vi "GetFovRayData.vi"(6 "Sensor position":cluster{"X":sgl, "Y":sgl, "Z":sgl}={"X"=0.0, "Y"=0.0, "Z"=70.75}, 8 "Max distance":dbl, 9 "Kinect FOV (deg)":cluster{"Height":i32, "Width":i32}, 10 "Sensor Yaw angle (deg)":dbl, 11 "Elevation Angle":i32) -> (3 "Planes":T1)   [LabVIEW 2014]
uses:
  <vilib>/Math Plots/3D Math Plots/3D Scatter/3D Scatter XCtrl/3D Scatter.xctl
  <vilib>/Math Plots/3D Math Plots/3D Plot/3D Plot Datatype/3D Plot Datatype.lvclass
  <vilib>/Math Plots/3D Math Plots/3D Scatter/3D Scatter Datatype/Public/Plot Helper (Vector).vi
  <vilib>/Analysis/coordinate.llb/3D Coordinate Conversion (Array).vi
  <vilib>/Analysis/NI_AALPro.lvlib
  <vilib>/Math Plots/3D Math Plots/3D Scatter/3D Scatter Datatype/3D Scatter Datatype.lvclass
panel:
  out "3D Scatter":refnum<class "3D Plot Datatype.lvclass">[](xcontrol)
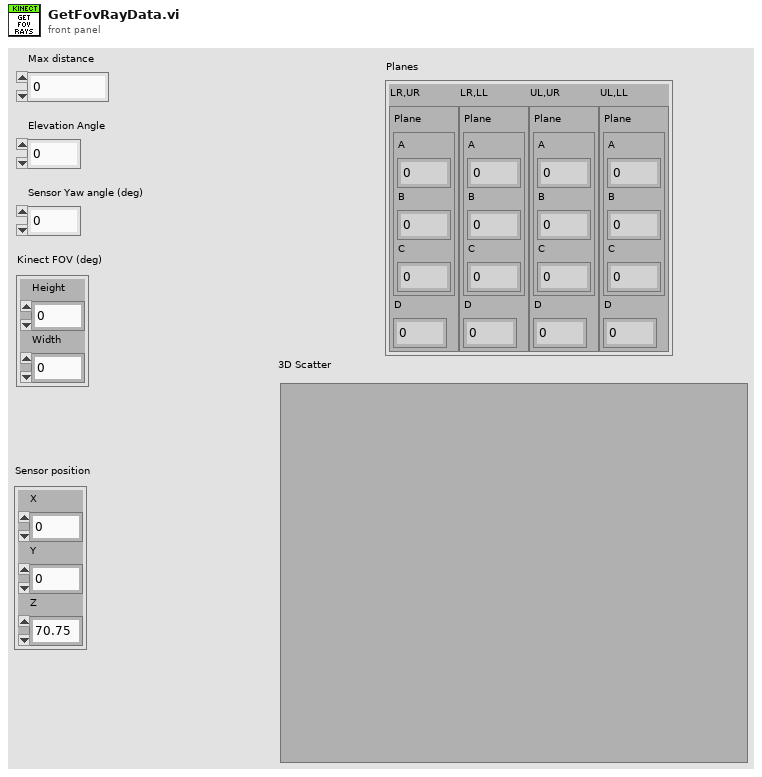
[diagram p1: front panel]
types:
  T1 = cluster{"LR,UR":cluster{"Plane":cluster{"A":dbl, "B":dbl, "C":dbl}, "D":dbl}, "LR,LL":cluster{"Plane":cluster{"A":dbl, "B":dbl, "C":dbl}, "D":dbl}, "UL,UR":cluster{"Plane":cluster{"A":dbl, "B":dbl, "C":dbl}, "D":dbl}, "UL,LL":cluster{"Plane":cluster{"A":dbl, "B":dbl, "C":dbl}, "D":dbl}}
  T2 = cluster{"Numeric":dbl, "Numeric":dbl, "Numeric":dbl}[]
  T3 = cluster{"Numeric":dbl, "Numeric":dbl, "Numeric":dbl}
  T4 = cluster{"Sensor position":cluster{"X":sgl, "Y":sgl, "Z":sgl}, cluster{"Numeric":dbl, "Numeric":dbl, "Numeric":dbl}, cluster{"Numeric":dbl, "Numeric":dbl, "Numeric":dbl}}
  T5 = cluster{"Plane":cluster{"A":dbl, "B":dbl, "C":dbl}, "D":dbl}
  T6 = cluster{"[0]":cluster{"Plane":cluster{"A":dbl, "B":dbl, "C":dbl}, "D":dbl}, "[1]":cluster{"Plane":cluster{"A":dbl, "B":dbl, "C":dbl}, "D":dbl}, "[2]":cluster{"Plane":cluster{"A":dbl, "B":dbl, "C":dbl}, "D":dbl}, "[3]":cluster{"Plane":cluster{"A":dbl, "B":dbl, "C":dbl}, "D":dbl}}
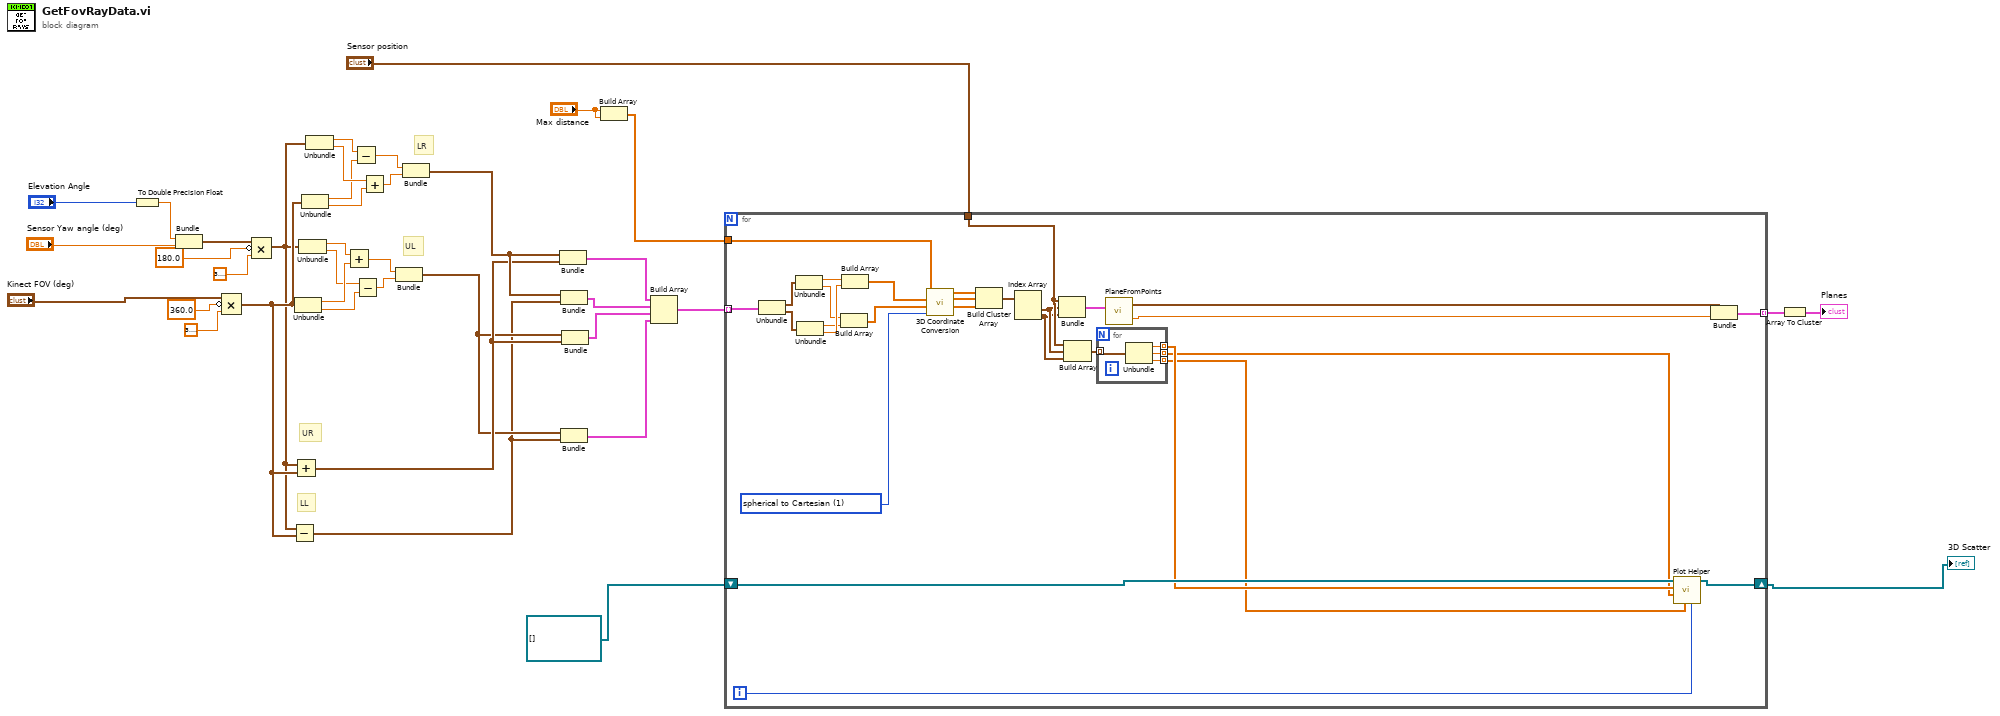
[diagram p0: block diagram]
diagram:
  # "LL"
  # "UR"
  # "UL"
  # "LR"
  n1 = To Double Precision Float(number="Elevation Angle") -> (double precision float=w37:dbl)
  n2 = Bundle(w37, "Sensor Yaw angle (deg)"="Sensor Yaw angle (deg)") -> (w36:cluster{dbl, "Sensor Yaw angle (deg)":dbl})  [unwired: 1 in]
  n3 = Compound Arithmetic op=MULTIPLY("Kinect FOV (deg)", invert 360.0 ("value"), 3.141592653589793) -> (w18:cluster{"Height":dbl, "Width":dbl})
  n4 = Compound Arithmetic op=MULTIPLY(w36, invert 180.0 ("value"), 3.141592653589793) -> (w17:cluster{dbl, "Sensor Yaw angle (deg)":dbl})
  n5 = Subtract(x=w17, y=w18) -> (x-y=w13:cluster{dbl, dbl})
  n6 = Add(x=w17, y=w18) -> (x+y=w15:cluster{dbl, dbl})
  n7 = Unbundle(w18) -> ("Height"=w29:dbl, "Width"=w27:dbl)
  n8 = Unbundle(w17) -> (w30:dbl, "Sensor Yaw angle (deg)"=w28:dbl)
  n9 = Unbundle(w18) -> ("Height"=w20:dbl, "Width"=w22:dbl)
  n10 = Unbundle(w17) -> (w19:dbl, "Sensor Yaw angle (deg)"=w21:dbl)
  n11 = Add(x=w30, y=w29) -> (x+y=w25:dbl)
  n12 = Subtract(x=w19, y=w20) -> (x-y=w24:dbl)
  n13 = Subtract(x=w28, y=w27) -> (x-y=w26:dbl)
  n14 = Add(x=w21, y=w22) -> (x+y=w23:dbl)
  n15 = Bundle(w25, w26) -> (w14:cluster{dbl, dbl})  [unwired: 1 in]
  n16 = Bundle(w24, w23) -> (w16:cluster{dbl, dbl})  [unwired: 1 in]
  n17 = Bundle(w16, w15) -> (w12:cluster{cluster{dbl, dbl}, cluster{dbl, dbl}})  [unwired: 1 in]
  n18 = Bundle(w16, w13) -> (w11:cluster{cluster{dbl, dbl}, cluster{dbl, dbl}})  [unwired: 1 in]
  n19 = Bundle(w14, w13) -> (w10:cluster{cluster{dbl, dbl}, cluster{dbl, dbl}})  [unwired: 1 in]
  n20 = Bundle(w14, w15) -> (w9:cluster{cluster{dbl, dbl}, cluster{dbl, dbl}})  [unwired: 1 in]
  n21 = Build Array("Max distance", "Max distance") -> (w6:dbl[])
  n22 = Build Array(w12, w11, w9, w10) -> (w8:cluster{cluster{dbl, dbl}, cluster{dbl, dbl}}[])
  n23 = for {
    tunnel: w8 -> [w67] mode=indexing
    tunnel: w6 -> [w60]
    tunnel: "Sensor position" -> [w53]
    tunnel: [w57] -> w4 mode=indexing
    shift-right: [w46] -> w1
    shift-left: refnum<class "3D Plot Datatype.lvclass">[] [] ("3D Plot lvclass Array out") -> [w47]
    i -> [w42]
    w68 = u16 1 items=["Cartesian to spherical", "spherical to Cartesian", "Cartesian to cylindrical", "cylindrical to Cartesian", "spherical to cylindrical", "cylindrical to spherical"] ("conversion type")
    n24 = Unbundle(w67) -> (w66:cluster{dbl, dbl}, w65:cluster{dbl, dbl})
    n25 = Unbundle(w66) -> (w64:dbl, w61:dbl)
    n26 = Unbundle(w65) -> (w62:dbl, w63:dbl)
    n27 = Build Array(w61, w62) -> (w40:dbl[])
    n28 = Build Array(w64, w63) -> (w41:dbl[])
    n29 = call-poly <vilib>:"3D Coordinate Conversion.vi"("conversion type"=w68, "Axis 3"=w40, "Axis 2"=w41, "Axis 1"=w60) -> ("Axis 3 Out"=w54:dbl[], "Axis 2 Out"=w56:dbl[], "Axis 1 Out"=w55:dbl[])  [unwired: 4 in, 1 out]
    n30 = Build Cluster Array(w55, w56, w54) -> (w59:T2)
    n31 = Index Array(array=w59) -> (element #1=w52:T3, element #2=w51:T3)  [unwired: 2 in]
    n32 = Bundle("Sensor position"=w53, w52, w51) -> (w58:T4)  [unwired: 1 in]
    n33 = Build Array(w53, w52, w51) -> (w50:T2)
    n34 = for {
      tunnel: w50 -> [w72] mode=indexing
      tunnel: [w71] -> w45 mode=indexing
      tunnel: [w70] -> w44 mode=indexing
      tunnel: [w69] -> w43 mode=indexing
      n35 = Unbundle(w72) -> ("Numeric"=w71:dbl, "Numeric"=w70:dbl, "Numeric"=w69:dbl)
    }
    n36 = call "PlaneFromPoints.vi"("Points"=w58) -> ("D"=w49:dbl, "Plane"=w48:cluster{"A":dbl, "B":dbl, "C":dbl})  [unwired: 1 in]
    n37 = call-poly <vilib>:"Plot Helper.vi"("Plot ID"=w42, "z vector"=w43, "y vector"=w44, "x vector"=w45, "3D Plot lvclass Array in"=w47) -> ("3D Plot lvclass Array out"=w46:refnum<class "3D Plot Datatype.lvclass">[])  [unwired: 1 in, 5 out]
    n38 = Bundle("Plane"=w48, "D"=w49) -> (w57:T5)  [unwired: 1 in]
  }
  "3D Scatter" <- w1
  n39 = Array To Cluster(array=w4) -> (cluster=→"Planes":T6)
